vi "Load Help File.vi"(8 "error in (no error)":errorcluster, 9 "HTML File to Load":string="MainPage_J1939.html", 11 "Browser":refnum<k7>(container)) -> (0 "error out":errorcluster)   [LabVIEW 2027, in "System Monitor System Explorer.lvlib"]
doc: "Loads the specified HTML page from the CHM into the browser"
uses:
  System Monitor System Explorer.lvlib
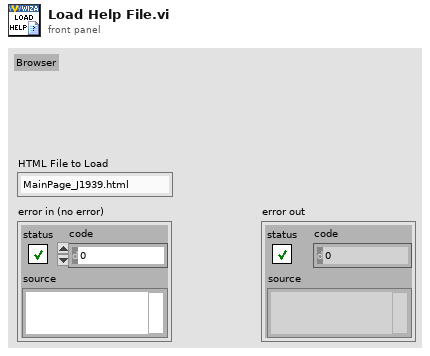
[diagram p1: front panel]
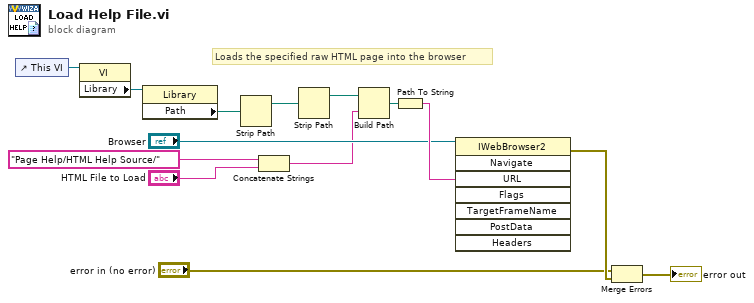
[diagram p0: block diagram]
diagram:
  # "Loads the specified raw HTML page into the browser"
  n1 = control-ref of="This VI"() -> (w7:refnum<vi>)
  n2 = property class="VI"(reference=w7) -> ("Library"=w6:refnum<vi>)  [unwired: 1 in, 2 out]
  n3 = property class="Library"(reference=w6) -> ("Path"=w2:path)  [unwired: 1 in, 2 out]
  n4 = Strip Path(path=w2) -> (stripped path=w3:path)  [unwired: 1 out]
  n5 = Concatenate Strings("Page Help/HTML Help Source/" ("name or relative path"), "HTML File to Load") -> (w1:string)
  n6 = Strip Path(path=w3) -> (stripped path=w5:path)  [unwired: 1 out]
  n7 = Build Path(base path=w5, name or relative path=w1) -> (appended path=w13:path)
  n8 = Path To String(path=w13) -> (string=w14:string)
  n9 = invoke class="IWebBrowser2" method="Navigate"(reference="Browser", "URL"=w14) -> (error out=w10:errorcluster)  [unwired: 6 in, 7 out]
  n10 = Merge Errors("error in (no error)", w10) -> (→"error out":errorcluster)
